vi "DG535.ProcEvents.vi"(0 "i ref in":refnum<vi>, 5 "error in":errorcluster) -> (14 "i ref out":refnum<vi>, 19 "error out":errorcluster)   [LabVIEW 2014, in "DG535.lvlib"]
doc: "This method is used to define the events the object will listen to. Add your own events here."
uses:
  DG535.lvlib
  CSCore/BaseProcess/BaseProcess.event definition.ctl
  CSCore/CAEObj/CAEObj.event definition.ctl
  CSCore/BaseProcess/BaseProcess.descriptor string definition.ctl
  CSCore/BaseProcess/BaseProcess.lvlib
  CSCore/CAEObj/CAEObj.lvlib
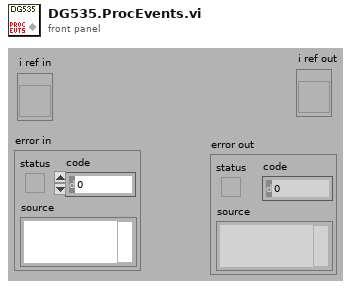
[diagram p1: front panel]
types:
  T1 = typedef "BaseProcess.lvlib/BaseProcess.event definition.ctl" = cluster{"CAEEvtDef":T2, "Data Descriptor":T3}
  T2 = typedef "CAEObj.lvlib/CAEObj.event definition.ctl" = cluster{"URL":string, "enable":bool, "ignoreResID":bool}
  T3 = typedef "BaseProcess.lvlib/BaseProcess.descriptor string definition.ctl" = string
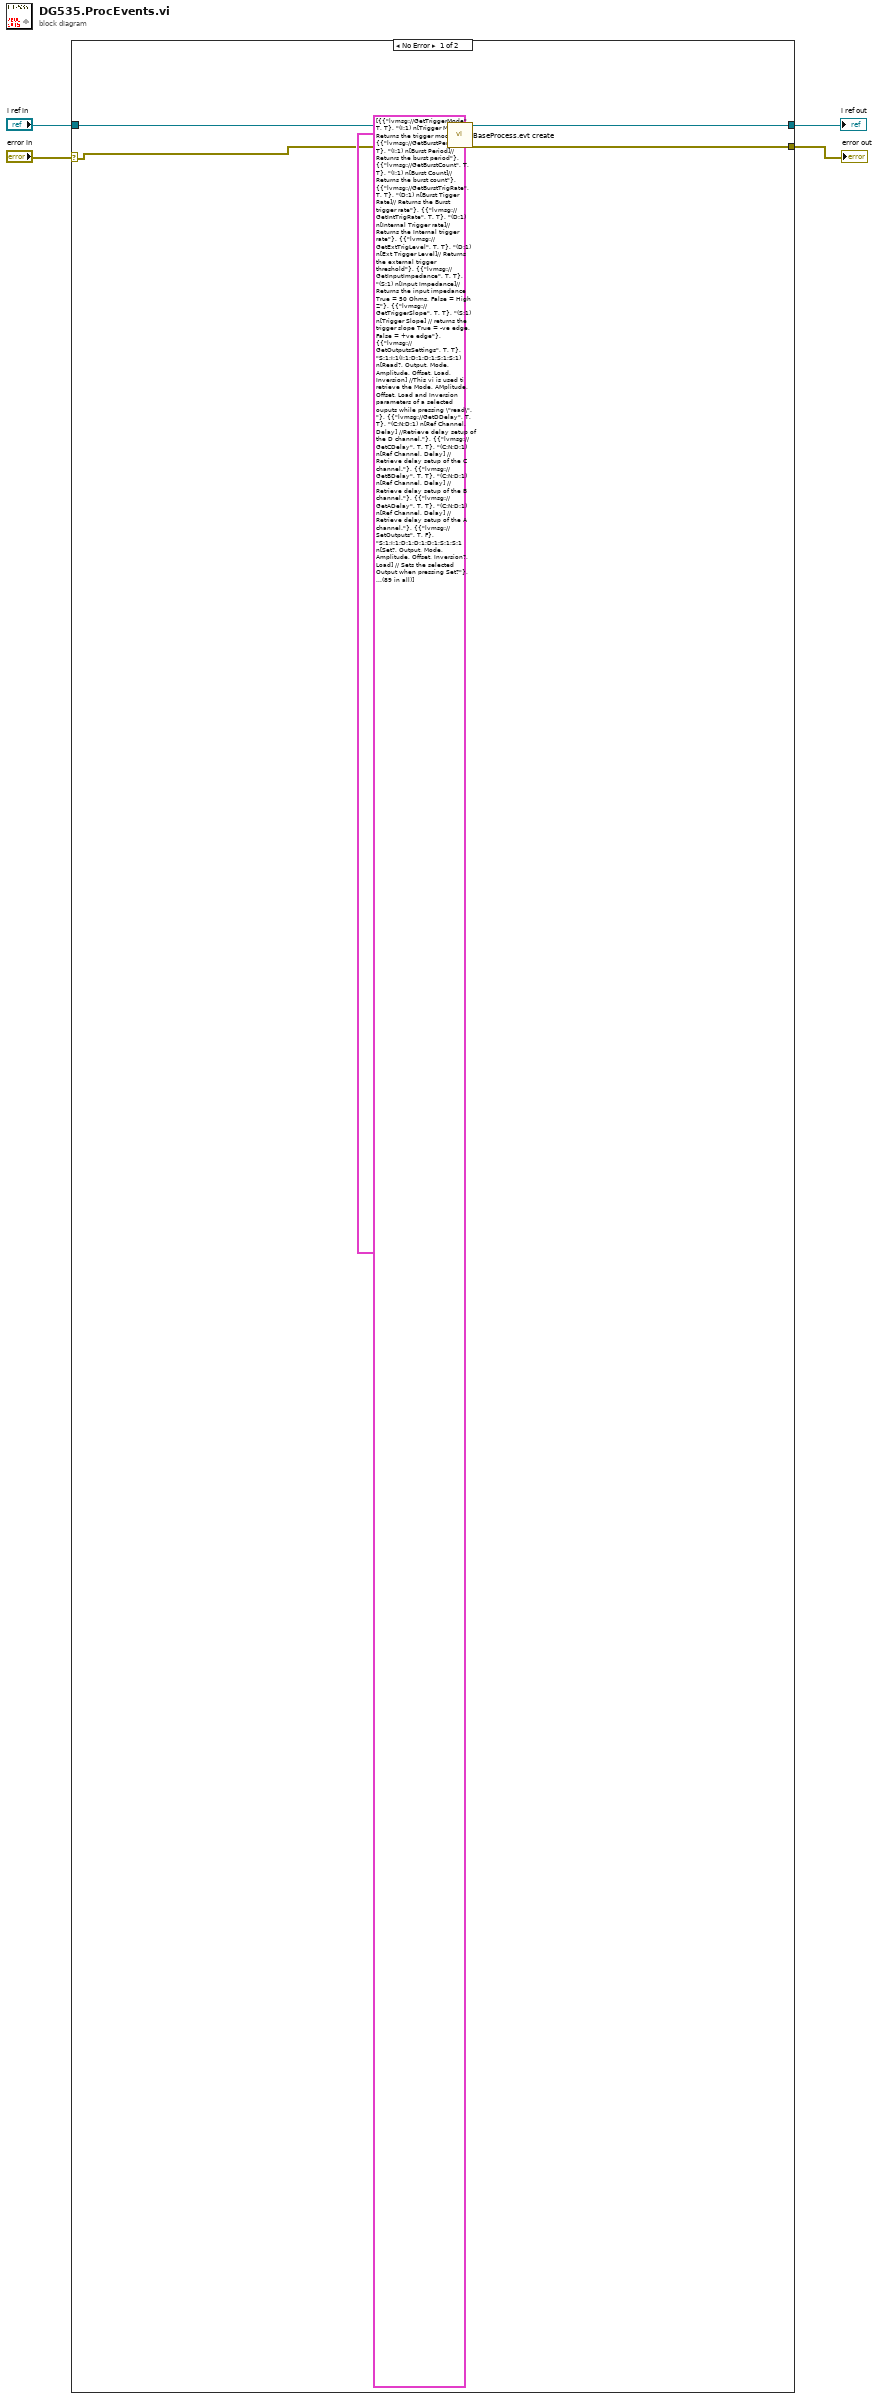
[diagram p0: block diagram]
diagram:
  n1 = case shown="No Error" "error in" {
    selector: "error in" -> [w5 w11]
    tunnel: "i ref in" -> [w9 w10]
    tunnel: [w8 w10] -> w3
    tunnel: [w7 w11] -> w2
    frame No Error {
      n2 = call "BaseProcess.evt create.vi"("i ref in"=w9, "newEvents"=T1[] [{"CAEEvtDef"={"URL"="lvmsg://GetTriggerMode", "enable"=TRUE, "ignoreResID"=TRUE}, "Data Descriptor"="(I:1) n[Trigger Mode]// Returns the trigger mode"}, {"CAEEvtDef"={"URL"="lvmsg://GetBurstPeriod", "enable"=TRUE, "ignoreResID"=TRUE}, "Data Descriptor"="(I:1) n[Burst Period]// Retunrs the burst period"}, {"CAEEvtDef"={"URL"="lvmsg://GetBurstCount", "enable"=TRUE, "ignoreResID"=TRUE}, "Data Descriptor"="(I:1) n[Burst Count]// Returns the burst count"}, {"CAEEvtDef"={"URL"="lvmsg://GetBurstTrigRate", "enable"=TRUE, "ignoreResID"=TRUE}, "Data Descriptor"="(D:1) n[Burst Tigger Rate]// Returns the Burst trigger rate"}, {"CAEEvtDef"={"URL"="lvmsg://GetIntTrigRate", "enable"=TRUE, "ignoreResID"=TRUE}, "Data Descriptor"="(D:1) n[Internal Trigger rate]// Returns the Internal trigger rate"}, {"CAEEvtDef"={"URL"="lvmsg://GetExtTrigLevel", "enable"=TRUE, "ignoreResID"=TRUE}, "Data Descriptor"="(D:1) n[Ext Trigger Level]// Returns the external trigger threshold"}, {"CAEEvtDef"={"URL"="lvmsg://GetInputImpedance", "enable"=TRUE, "ignoreResID"=TRUE}, "Data Descriptor"="(S:1) n[Input Impedance]// Returns the input impedance True = 50 Ohms, False = High Z"}, {"CAEEvtDef"={"URL"="lvmsg://GetTriggerSlope", "enable"=TRUE, "ignoreResID"=TRUE}, "Data Descriptor"="(S:1) n[Trigger Slope] // returns the trigger slope True = -ve edge, False = +ve edge"}, {"CAEEvtDef"={"URL"="lvmsg://GetOutputsSettings", "enable"=TRUE, "ignoreResID"=TRUE}, "Data Descriptor"="S:1;I:1(I:1;D:1;D:1;S:1;S:1) n[Read?, Output, Mode, Amplitude, Offset, Load, Inversion] //This vi is used ti retrieve the Mode, AMplitude, Offset, Load and Inversion parameters of a selected ouputs while pressing \"read\"."}, {"CAEEvtDef"={"URL"="lvmsg://GetDDelay", "enable"=TRUE, "ignoreResID"=TRUE}, "Data Descriptor"="(C:N;D:1) n[Ref Channel, Delay] //Retrieve delay setup of the D channel."}, {"CAEEvtDef"={"URL"="lvmsg://GetCDelay", "enable"=TRUE, "ignoreResID"=TRUE}, "Data Descriptor"="(C:N;D:1) n[Ref Channel, Delay] //Retrieve delay setup of the C channel."}, {"CAEEvtDef"={"URL"="lvmsg://GetBDelay", "enable"=TRUE, "ignoreResID"=TRUE}, "Data Descriptor"="(C:N;D:1) n[Ref Channel, Delay] //Retrieve delay setup of the B channel."}, {"CAEEvtDef"={"URL"="lvmsg://GetADelay", "enable"=TRUE, "ignoreResID"=TRUE}, "Data Descriptor"="(C:N;D:1) n[Ref Channel, Delay] //Retrieve delay setup of the A channel."}, {"CAEEvtDef"={"URL"="lvmsg://SetOutputs", "enable"=TRUE, "ignoreResID"=FALSE}, "Data Descriptor"="S:1;I:1;D:1;D:1;D:1;S:1;S:1 n[Set?, Output, Mode, Amplitude, Offset, Inversion?, Load] // Sets the selected Output when pressing Set?"}, {"CAEEvtDef"={"URL"="lvmsg://SetDelays", "enable"=TRUE, "ignoreResID"=FALSE}, "Data Descriptor"="I:1;D:1;I:1;D:1;I:1;D:1;I:1;D:1 n[A ref, A delay, B ref, B delay, C ref, C delay, D ref, D delay] // Sets delay A, B, C and D in a row."}, {"CAEEvtDef"={"URL"="lvmsg://GetCDMode", "enable"=TRUE, "ignoreResID"=TRUE}, "Data Descriptor"="(I:1) n[CD Mode] //Sets the channel CD mode : TTL, NIM, ECL, VARiable."}, {"CAEEvtDef"={"URL"="lvmsg://GetDMode", "enable"=TRUE, "ignoreResID"=TRUE}, "Data Descriptor"="(I:1) n[D Mode] //Sets the channel D mode : TTL, NIM, ECL, VARiable."}, {"CAEEvtDef"={"URL"="lvmsg://GetCMode", "enable"=TRUE, "ignoreResID"=TRUE}, "Data Descriptor"="(I:1) n[C Mode] //Sets the channel C mode : TTL, NIM, ECL, VARiable."}, {"CAEEvtDef"={"URL"="lvmsg://GetABMode", "enable"=TRUE, "ignoreResID"=TRUE}, "Data Descriptor"="(I:1) n[AB Mode] //Sets the channel AB mode : TTL, NIM, ECL, VARiable."}, {"CAEEvtDef"={"URL"="lvmsg://GetBMode", "enable"=TRUE, "ignoreResID"=TRUE}, "Data Descriptor"="(I:1) n[B Mode] //Sets the channel B mode : TTL, NIM, ECL, VARiable."}, {"CAEEvtDef"={"URL"="lvmsg://GetAMode", "enable"=TRUE, "ignoreResID"=TRUE}, "Data Descriptor"="(I:1) n[A Mode] //Sets the channel A mode : TTL, NIM, ECL, VARiable."}, {"CAEEvtDef"={"URL"="lvmsg://GetT0Mode", "enable"=TRUE, "ignoreResID"=TRUE}, "Data Descriptor"="(I:1) n[T0 Mode] //Sets the channel T0 mode : TTL, NIM, ECL, VARiable."}, {"CAEEvtDef"={"URL"="lvmsg://GetCDOffset", "enable"=TRUE, "ignoreResID"=TRUE}, "Data Descriptor"="(D:1) n[CD Offset] // Returns the CD channel offset."}, {"CAEEvtDef"={"URL"="lvmsg://GetDOffset", "enable"=TRUE, "ignoreResID"=TRUE}, "Data Descriptor"="(D:1) n[D Offset] // Returns the D channel offset."}, {"CAEEvtDef"={"URL"="lvmsg://GetCOffset", "enable"=TRUE, "ignoreResID"=TRUE}, "Data Descriptor"="(D:1) n[C Offset] // Returns the C channel offset."}, {"CAEEvtDef"={"URL"="lvmsg://GetABOffset", "enable"=TRUE, "ignoreResID"=TRUE}, "Data Descriptor"="(D:1) n[AB Offset] // Returns the AB channel offset."}, {"CAEEvtDef"={"URL"="lvmsg://GetBOffset", "enable"=TRUE, "ignoreResID"=TRUE}, "Data Descriptor"="(D:1) n[B Offset] // Returns the B channel offset."}, {"CAEEvtDef"={"URL"="lvmsg://GetAOffset", "enable"=TRUE, "ignoreResID"=TRUE}, "Data Descriptor"="(D:1) n[A Offset] // Returns the A channel offset."}, {"CAEEvtDef"={"URL"="lvmsg://GetT0Offset", "enable"=TRUE, "ignoreResID"=TRUE}, "Data Descriptor"="(D:1) n[T0 Offset] // Returns the T0 channel offset."}, {"CAEEvtDef"={"URL"="lvmsg://GetCDAmplitude", "enable"=TRUE, "ignoreResID"=TRUE}, "Data Descriptor"="(D:1) n[CD Amplitude] // Returns the CD channel amplitude."}, {"CAEEvtDef"={"URL"="lvmsg://GetDAmplitude", "enable"=TRUE, "ignoreResID"=TRUE}, "Data Descriptor"="(D:1) n[D Amplitude] // Returns the D channel amplitude."}, {"CAEEvtDef"={"URL"="lvmsg://GetCAmplitude", "enable"=TRUE, "ignoreResID"=TRUE}, "Data Descriptor"="(D:1) n[C Amplitude] // Returns the C channel amplitude."}, {"CAEEvtDef"={"URL"="lvmsg://GetABAmplitude", "enable"=TRUE, "ignoreResID"=TRUE}, "Data Descriptor"="(D:1) n[AB Amplitude] // Returns the AB channel amplitude."}, {"CAEEvtDef"={"URL"="lvmsg://GetBAmplitude", "enable"=TRUE, "ignoreResID"=TRUE}, "Data Descriptor"="(D:1) n[B Amplitude] // Returns the B channel amplitude."}, {"CAEEvtDef"={"URL"="lvmsg://GetAAmplitude", "enable"=TRUE, "ignoreResID"=TRUE}, "Data Descriptor"="(D:1) n[A Amplitude] // Returns the A channel amplitude."}, {"CAEEvtDef"={"URL"="lvmsg://GetT0Amplitude", "enable"=TRUE, "ignoreResID"=TRUE}, "Data Descriptor"="(D:1) n[T0 Amplitude] // Returns the T0 channel amplitude."}, {"CAEEvtDef"={"URL"="lvmsg://GetCDPolarity", "enable"=TRUE, "ignoreResID"=TRUE}, "Data Descriptor"="(S:1) n[CD Polarity] // Returns the channel AB Polarity, True= -, False=+."}, {"CAEEvtDef"={"URL"="lvmsg://GetABPolarity", "enable"=TRUE, "ignoreResID"=TRUE}, "Data Descriptor"="(S:1) n[AB Polarity] // Returns the channel AB Polarity, True= -, False=+."}, {"CAEEvtDef"={"URL"="lvmsg://GetCDLoad", "enable"=TRUE, "ignoreResID"=TRUE}, "Data Descriptor"="(S:1) n[CD Load] // Gets the Load status off the CD channel, True=50 Ohms, False=High Z."}, {"CAEEvtDef"={"URL"="lvmsg://GetDLoad", "enable"=TRUE, "ignoreResID"=TRUE}, "Data Descriptor"="(S:1) n[D Load] // Gets the Load status off the D channel, True=50 Ohms, False=High Z."}, {"CAEEvtDef"={"URL"="lvmsg://GetCLoad", "enable"=TRUE, "ignoreResID"=TRUE}, "Data Descriptor"="(S:1) n[C Load] // Gets the Load status off the C channel, True=50 Ohms, False=High Z."}, {"CAEEvtDef"={"URL"="lvmsg://GetABLoad", "enable"=TRUE, "ignoreResID"=TRUE}, "Data Descriptor"="(S:1) n[AB Load] // Gets the Load status off the AB channel, True=50 Ohms, False=High Z."}, {"CAEEvtDef"={"URL"="lvmsg://GetBLoad", "enable"=TRUE, "ignoreResID"=TRUE}, "Data Descriptor"="(S:1) n[B Load] // Gets the Load status off the B channel, True=50 Ohms, False=High Z."}, {"CAEEvtDef"={"URL"="lvmsg://GetALoad", "enable"=TRUE, "ignoreResID"=TRUE}, "Data Descriptor"="(S:1) n[A Load] // Gets the Load status off the A channel, True=50 Ohms, False=High Z."}, {"CAEEvtDef"={"URL"="lvmsg://GetT0Load", "enable"=TRUE, "ignoreResID"=TRUE}, "Data Descriptor"="(S:1) n[T0 Load] // Gets the Load status off the T0 channel, True=50 Ohms, False=High Z."}, {"CAEEvtDef"={"URL"="lvmsg://SetDDelay", "enable"=TRUE, "ignoreResID"=FALSE}, "Data Descriptor"="C:N;D:1 n[Reference Channel, D Delay] // Defines A delay by chosing reference and offset."}, {"CAEEvtDef"={"URL"="lvmsg://SetCDelay", "enable"=TRUE, "ignoreResID"=FALSE}, "Data Descriptor"="C:N;D:1 n[Reference Channel, C Delay] // Defines A delay by chosing reference and offset."}, {"CAEEvtDef"={"URL"="lvmsg://SetBDelay", "enable"=TRUE, "ignoreResID"=FALSE}, "Data Descriptor"="C:N;D:1 n[Reference Channel, B Delay] // Defines A delay by chosing reference and offset."}, {"CAEEvtDef"={"URL"="lvmsg://SetADelay", "enable"=TRUE, "ignoreResID"=FALSE}, "Data Descriptor"="C:N;D:1 n[Reference Channel, A Delay] // Defines A delay by chosing reference and offset."}, {"CAEEvtDef"={"URL"="lvmsg://SetCDLoad", "enable"=TRUE, "ignoreResID"=FALSE}, "Data Descriptor"="S:1 n[CD Load]// Defines the the channel CD load, High Z or 50 Ohms."}, {"CAEEvtDef"={"URL"="lvmsg://SetDLoad", "enable"=TRUE, "ignoreResID"=FALSE}, "Data Descriptor"="S:1 n[D Load]// Defines the the channel D load, High Z or 50 Ohms."}, {"CAEEvtDef"={"URL"="lvmsg://SetCLoad", "enable"=TRUE, "ignoreResID"=FALSE}, "Data Descriptor"="S:1 n[C Load]// Defines the the channel C load, High Z or 50 Ohms."}, {"CAEEvtDef"={"URL"="lvmsg://SetABLoad", "enable"=TRUE, "ignoreResID"=FALSE}, "Data Descriptor"="S:1 n[AB Load]// Defines the the channel AB load, High Z or 50 Ohms."}, {"CAEEvtDef"={"URL"="lvmsg://SetBLoad", "enable"=TRUE, "ignoreResID"=FALSE}, "Data Descriptor"="S:1 n[B Load]// Defines the the channel B load, High Z or 50 Ohms."}, {"CAEEvtDef"={"URL"="lvmsg://SetALoad", "enable"=TRUE, "ignoreResID"=FALSE}, "Data Descriptor"="S:1 n[A Load]// Defines the the channel A load, High Z or 50 Ohms."}, {"CAEEvtDef"={"URL"="lvmsg://SetT0Load", "enable"=TRUE, "ignoreResID"=FALSE}, "Data Descriptor"="S:1 n[T0 Load]// Defines the the channel T0 load, High Z or 50 Ohms."}, {"CAEEvtDef"={"URL"="lvmsg://SetCDOffset", "enable"=TRUE, "ignoreResID"=FALSE}, "Data Descriptor"="D:1 n[CD Offset] //Sets the channel CD Offset"}, {"CAEEvtDef"={"URL"="lvmsg://SetDOffset", "enable"=TRUE, "ignoreResID"=FALSE}, "Data Descriptor"="D:1 n[D Offset] //Sets the channel D Offset"}, {"CAEEvtDef"={"URL"="lvmsg://SetCOffset", "enable"=TRUE, "ignoreResID"=FALSE}, "Data Descriptor"="D:1 n[C Offset] //Sets the channel C Offset"}, {"CAEEvtDef"={"URL"="lvmsg://SetABOffset", "enable"=TRUE, "ignoreResID"=FALSE}, "Data Descriptor"="D:1 n[AB Offset] //Sets the channel AB Offset"}, {"CAEEvtDef"={"URL"="lvmsg://SetBOffset", "enable"=TRUE, "ignoreResID"=FALSE}, "Data Descriptor"="D:1 n[B Offset] //Sets the channel B Offset"}, {"CAEEvtDef"={"URL"="lvmsg://SetAOffset", "enable"=TRUE, "ignoreResID"=FALSE}, "Data Descriptor"="D:1 n[A Offset] //Sets the channel A Offset"}, {"CAEEvtDef"={"URL"="lvmsg://SetT0Offset", "enable"=TRUE, "ignoreResID"=FALSE}, "Data Descriptor"="D:1 n[T0 Offset] //Sets the channel T0 Offset"}, {"CAEEvtDef"={"URL"="lvmsg://SetCDAmplitude", "enable"=TRUE, "ignoreResID"=FALSE}, "Data Descriptor"="D:1 n[CD Amplitude] //Sets the channel CD Amplitude."}, {"CAEEvtDef"={"URL"="lvmsg://SetDAmplitude", "enable"=TRUE, "ignoreResID"=FALSE}, "Data Descriptor"="D:1 n[D Amplitude] //Sets the channel D Amplitude."}, {"CAEEvtDef"={"URL"="lvmsg://SetCAmplitude", "enable"=TRUE, "ignoreResID"=FALSE}, "Data Descriptor"="D:1 n[C Amplitude] //Sets the channel C Amplitude."}, {"CAEEvtDef"={"URL"="lvmsg://SetABAmplitude", "enable"=TRUE, "ignoreResID"=FALSE}, "Data Descriptor"="D:1 n[AB Amplitude] //Sets the channel AB Amplitude."}, {"CAEEvtDef"={"URL"="lvmsg://SetBAmplitude", "enable"=TRUE, "ignoreResID"=FALSE}, "Data Descriptor"="D:1 n[B Amplitude] //Sets the channel B Amplitude."}, {"CAEEvtDef"={"URL"="lvmsg://SetAAmplitude", "enable"=TRUE, "ignoreResID"=FALSE}, "Data Descriptor"="D:1 n[A Amplitude] //Sets the channel A Amplitude."}, {"CAEEvtDef"={"URL"="lvmsg://SetT0Amplitude", "enable"=TRUE, "ignoreResID"=FALSE}, "Data Descriptor"="D:1 n[T0 Amplitude] //Sets the channel T0 Amplitude."}, {"CAEEvtDef"={"URL"="lvmsg://SetCDInversion", "enable"=TRUE, "ignoreResID"=FALSE}, "Data Descriptor"="S:1 n[CD Inversion On/Off] // Switch channel CD inversion On/Off"}, {"CAEEvtDef"={"URL"="lvmsg://SetABInversion", "enable"=TRUE, "ignoreResID"=FALSE}, "Data Descriptor"="S:1 n[AB Inversion On/Off] // Switch channel AB inversion On/Off"}, {"CAEEvtDef"={"URL"="lvmsg://SetCDMode", "enable"=TRUE, "ignoreResID"=FALSE}, "Data Descriptor"="I:1 n[CD Mode] //Sets the channel CD mode : TTL, NIM, ECL, VARiable."}, {"CAEEvtDef"={"URL"="lvmsg://SetDMode", "enable"=TRUE, "ignoreResID"=FALSE}, "Data Descriptor"="I:1 n[D Mode] //Sets the channel D mode : TTL, NIM, ECL, VARiable."}, {"CAEEvtDef"={"URL"="lvmsg://SetCMode", "enable"=TRUE, "ignoreResID"=FALSE}, "Data Descriptor"="I:1 n[C Mode] //Sets the channel C mode : TTL, NIM, ECL, VARiable."}, {"CAEEvtDef"={"URL"="lvmsg://SetABMode", "enable"=TRUE, "ignoreResID"=FALSE}, "Data Descriptor"="I:1 n[AB Mode] //Sets the channel AB mode : TTL, NIM, ECL, VARiable."}, {"CAEEvtDef"={"URL"="lvmsg://SetBMode", "enable"=TRUE, "ignoreResID"=FALSE}, "Data Descriptor"="I:1 n[B Mode] //Sets the channel B mode : TTL, NIM, ECL, VARiable."}, {"CAEEvtDef"={"URL"="lvmsg://SetAMode", "enable"=TRUE, "ignoreResID"=FALSE}, "Data Descriptor"="I:1 n[A Mode] //Sets the channel A mode : TTL, NIM, ECL, VARiable."}, {"CAEEvtDef"={"URL"="lvmsg://SetT0Mode", "enable"=TRUE, "ignoreResID"=FALSE}, "Data Descriptor"="I:1 n[T0 Mode] //Sets the channel T0 mode : TTL, NIM, ECL, VARiable."}, {"CAEEvtDef"={"URL"="lvmsg://SetInputImpedance", "enable"=TRUE, "ignoreResID"=FALSE}, "Data Descriptor"="S:1 n[Input Impedance]// Defines the the Input Impedance, High Z or 50 Ohms."}, {"CAEEvtDef"={"URL"="lvmsg://SetTriggerSlope", "enable"=TRUE, "ignoreResID"=FALSE}, "Data Descriptor"="S:1 n[Input Impedance]// Defines the the Input Impedance, High Z or 50 Ohms."}, {"CAEEvtDef"={"URL"="lvmsg://SetExtTrigLvl", "enable"=TRUE, "ignoreResID"=FALSE}, "Data Descriptor"="D:1 n[External Trigger Level] // Sets the external trigger level."}, {"CAEEvtDef"={"URL"="lvmsg://SetBurstCount", "enable"=TRUE, "ignoreResID"=FALSE}, "Data Descriptor"="I:1 n[Burst Count] //Sets the number of pulses which will be in each burst of pulses."}, {"CAEEvtDef"={"URL"="lvmsg://SetBurstPeriod", "enable"=TRUE, "ignoreResID"=FALSE}, "Data Descriptor"="I:1 n[Burst Period] // Sets the number of triggers between the start of each burst of pulses when in the burst mode."}, {"CAEEvtDef"={"URL"="lvmsg://SetBurstTrigRate", "enable"=TRUE, "ignoreResID"=FALSE}, "Data Descriptor"="D:1 n[Burst Trigger Rate] // Sets the burst trigger rate."}, {"CAEEvtDef"={"URL"="lvmsg://SetInternalTrigRate", "enable"=TRUE, "ignoreResID"=FALSE}, "Data Descriptor"="D:1 n[Internal Trigger Rate] // Sets the internal trigger rate."}, {"CAEEvtDef"={"URL"="lvmsg://SetTriggerMode", "enable"=TRUE, "ignoreResID"=FALSE}, "Data Descriptor"="I:1 n[Trigger Mode] // Defines the Trigger Mode: Internal, External, Single Shot or Burst."}, {"CAEEvtDef"={"URL"="lvmsg://SetDelay", "enable"=TRUE, "ignoreResID"=FALSE}, "Data Descriptor"="D:1 n[A Delay] //sets delay time in micro seconds"}, {"CAEEvtDef"={"URL"="lvmsg://GetActDelay", "enable"=TRUE, "ignoreResID"=TRUE}, "Data Descriptor"="(D:1) n[Actdelay {us}] //Gets the Delay that has been set recently (-1 if error)"}] ("new events"), "error in (no error)"=w5) -> ("i ref out"=w8:refnum<vi>, "error out"=w7:errorcluster)  [unwired: 13 in, 2 out]
    }
    frame Error {
    }
  }
  "i ref out" <- w3
  "error out" <- w2
